vi "RP100SetVoltage.vi"(2 "error in (no error)":errorcluster, 3 "Voltage":dbl, 4 "Source":enum16{"1", "2", "Both"}(ring), 5 "VISA resource name":refnum<visa-resource-name>) -> (0 "error out":errorcluster, 1 "VISA resource name out":refnum<visa-resource-name>)   [LabVIEW 2019, in "RP100.lvlib"]
uses:
  RP100.lvlib
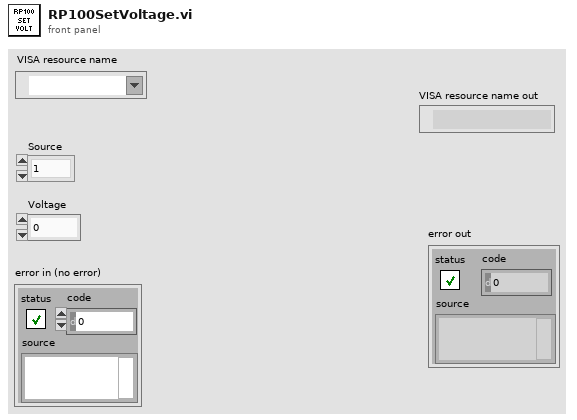
[diagram p1: front panel]
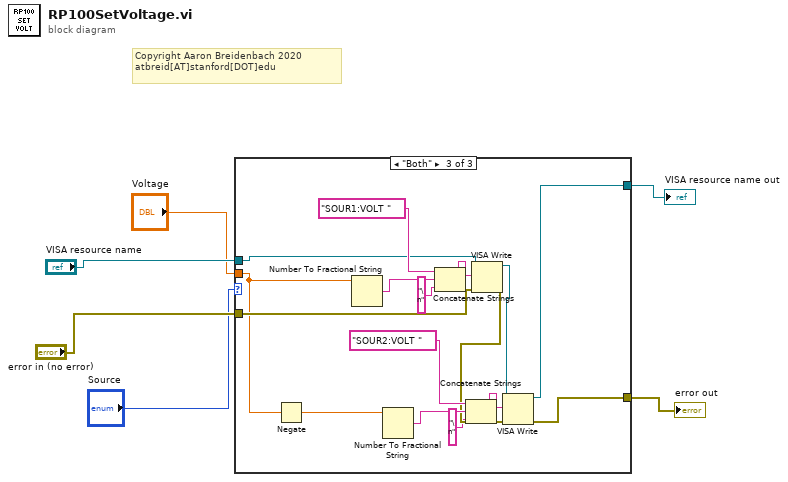
[diagram p0: block diagram]
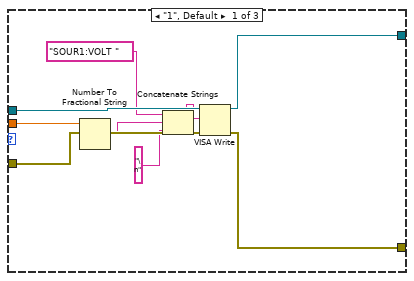
[diagram p2: hidden frame]
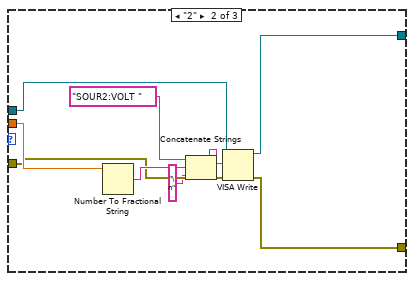
[diagram p3: hidden frame]
diagram:
  # "Copyright Aaron Breidenbach 2020\natbreid[AT]stanford[DOT]edu"
  n1 = case shown="\"Both\"" "Source" {
    tunnel: "VISA resource name" -> [w15 w18 w34]
    tunnel: "error in (no error)" -> [w14 w17 w31]
    tunnel: "Voltage" -> [w10 w19 w26]
    tunnel: [w7 w20 w32] -> w2
    tunnel: [w8 w21 w33] -> w1
    frame "1", Default {
      n2 = Number To Fractional String(number=w10) -> (F-format string=w12:string)  [unwired: 3 in]
      n3 = Concatenate Strings("SOUR1:VOLT " ("write buffer"), w12, "\n" ("string")) -> (w13:string)
      n4 = VISA Write(VISA resource name=w15, write buffer=w13, error in (no error)=w14) -> (VISA resource name out=w8:refnum<visa-resource-name>, error out=w7:errorcluster)  [unwired: 1 out]
    }
    frame "2" {
      n5 = Number To Fractional String(number=w19) -> (F-format string=w23:string)  [unwired: 3 in]
      n6 = Concatenate Strings("SOUR2:VOLT " ("write buffer"), w23, "\n" ("string")) -> (w24:string)
      n7 = VISA Write(VISA resource name=w18, write buffer=w24, error in (no error)=w17) -> (VISA resource name out=w21:refnum<visa-resource-name>, error out=w20:errorcluster)  [unwired: 1 out]
    }
    frame "Both" {
      n8 = Negate(x=w26) -> (-x=w25:dbl)
      n9 = Number To Fractional String(number=w26) -> (F-format string=w39:string)  [unwired: 3 in]
      n10 = Number To Fractional String(number=w25) -> (F-format string=w36:string)  [unwired: 3 in]
      n11 = Concatenate Strings("SOUR1:VOLT " ("write buffer"), w39, "\n" ("string")) -> (w40:string)
      n12 = Concatenate Strings("SOUR2:VOLT " ("write buffer"), w36, "\n" ("string")) -> (w37:string)
      n13 = VISA Write(VISA resource name=w34, write buffer=w40, error in (no error)=w31) -> (VISA resource name out=w30:refnum<visa-resource-name>, error out=w29:errorcluster)  [unwired: 1 out]
      n14 = VISA Write(VISA resource name=w30, write buffer=w37, error in (no error)=w29) -> (VISA resource name out=w33:refnum<visa-resource-name>, error out=w32:errorcluster)  [unwired: 1 out]
    }
  }
  "error out" <- w2
  "VISA resource name out" <- w1
